vi "cRIO_onboard_laser_log.vi"() -> ()   [LabVIEW 2020]
uses:
  <vilib>/Platform/TimedLoop/XDataNode/timing_clust.ctl
  <vilib>/Platform/TimedLoop/XDataNode/nitl_modes.ctl
  <vilib>/Platform/TimedLoop/XDataNode/wakeup.ctl
  <vilib>/Utility/file.llb/Write Delimited Spreadsheet (DBL).vi
  <vilib>/Platform/TimedLoop/XDataNode/loadnilvce.vi
  <vilib>/platform/TimedLoop/XDataNode/XDataNode.xnode
  <vilib>/Platform/TimedLoop/XDataNode/XDNodeRunTimeDep.lvlib
panel:
  out "Laser Displacement - cRIO (onboard execution)":dbl[][](graph)
  out "Readout (V)":dbl[][](array[numeric])
  in  "Log Data":bool
  out "Laser Displacement - cRIO (logged data)":dbl[][](graph)
  in  "stop":bool
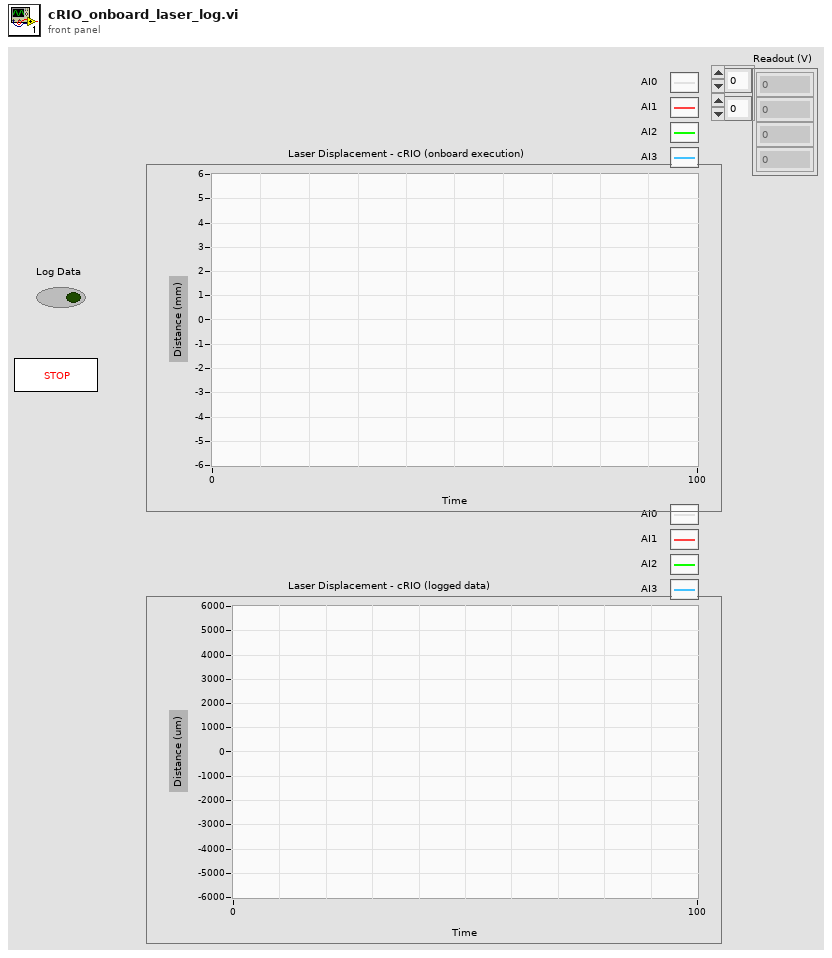
[diagram p1: front panel]
types:
  T1 = typedef "XDNodeRunTimeDep.lvlib/timing_clust.ctl" = cluster{"Expected End [f-1]":u64, "Actual End [f-1]":u64, "Finished Late? [f-1]":bool, "Expected End [i-1]":u64, "Actual End [i-1]":u64, "Finished Late? [i-1]":bool, "Expected Start [i]":u64, "Actual Start [i]":u64, "Expected Start [f]":u64, "Actual Start [f]":u64, "Source Name":string, "Structure Name":string, "Period":i64, "Deadline":i64, "Offset":i64, "Start":i64, "Priority":i32, "Timeout":i32, "Mode":T2, "Wakeup Reason":T3, "Error":errorcluster, "Source Type":string, "Secondary Source Type":string, "Global End Time":u64, "Global Start Time":u64, "Frame Duration":u64, "Iteration Duration":u64, "Assigned CPU":i32, "I/O Scan Engine Mode":u32}
  T2 = typedef "XDNodeRunTimeDep.lvlib/nitl_modes.ctl" = enum32{"No Change", "Process missed periods, maintain original phase", "Discard missed periods, maintain original phase", "Process missed periods, ignore original phase", "Discard missed periods, ignore original phase"}
  T3 = typedef "XDNodeRunTimeDep.lvlib/wakeup.ctl" = enum32{"Normal", "Aborted", "Asynchronous wakeup", "Timing source error", "Timed loop error", "Timeout"}
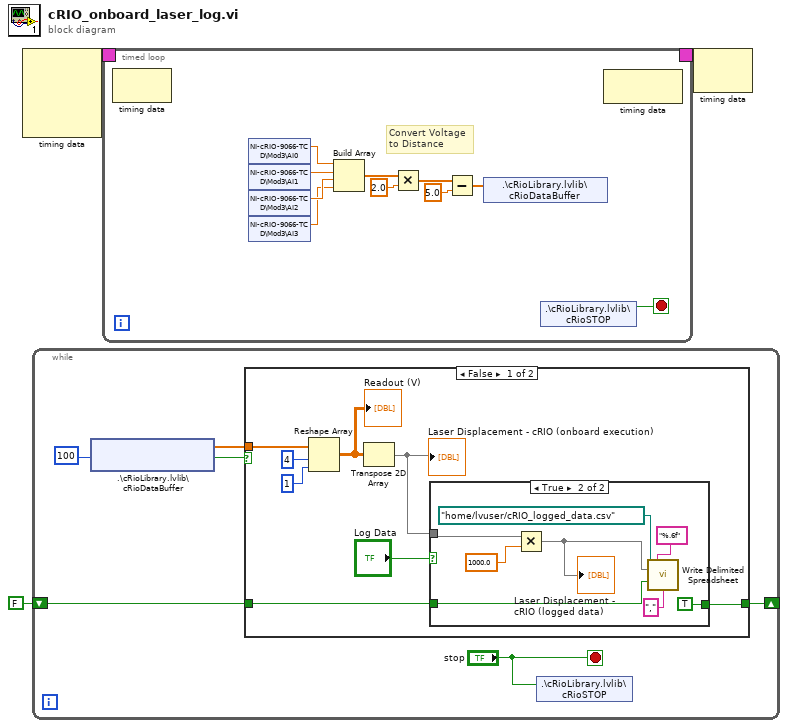
[diagram p0: block diagram]
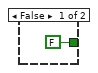
[diagram p2: hidden frame]
diagram:
  n1 = node-c288() -> (w3:T1)  [unwired: 4 in]
  n2 = while {
    shift-right: [w9] -> _
    shift-left: FALSE -> [w8]
    stop <- "stop" stop-if-true
    n3 = shared-variable ".\\cRioLibrary.lvlib\\cRioDataBuffer"(100) -> (w6:dbl[], w5:bool)  [unwired: 1 in, 1 out]
    n4 = case shown="False" w5 {
      tunnel: w6 -> [w11 _]
      tunnel: [w12 w27] -> w9
      tunnel: w8 -> [w17 w27]
      frame False {
        n5 = Reshape Array(w11, 4 ("dimension size"), 1 ("dimension size")) -> (w14:dbl[][])
        "Readout (V)" <- w14
        n6 = Transpose 2D Array(2D array=w14) -> (transposed array=w10:dbl[][])
        "Laser Displacement - cRIO (onboard execution)" <- w10
        n7 = case shown="True" "Log Data" {
          tunnel: w17 -> [_ w21]
          tunnel: w10 -> [_ w25]
          tunnel: [FALSE TRUE] -> w12
          frame False {
          }
          frame True {
            n8 = Multiply(x=w25, y=1000.0) -> (x*y=w19:dbl[][])
            "Laser Displacement - cRIO (logged data)" <- w19
            n9 = call-poly <vilib>:"Write Delimited Spreadsheet.vi"("file path (dialog if empty)"=path "/home/lvuser/cRIO_logged_data.csv", "format (%.3f)"="%.6f", "2D data"=w19, "append to file? (new file:F)"=w21, "delimiter (\\t)"="," ("delimiter (\\t)")) -> ()  [unwired: 9 in, 2 out]
          }
        }
      }
      frame True {
      }
    }
    n10 = shared-variable ".\\cRioLibrary.lvlib\\cRioSTOP"("stop") -> ()  [unwired: 1 in, 1 out]
  }
  n11 = timed-loop {
    timing: w3 -> [_]
    timing-out: [_] -> w2
    stop <- w37 stop-if-true
    # "Convert Voltage to Distance"
    n12 = node-c288() -> ()  [unwired: 1 in, 1 out]
    n13 = shared-variable "NI-cRIO-9066-TCD\\Mod3\\AI0"() -> (w33:dbl)  [unwired: 1 in, 1 out]
    n14 = shared-variable "NI-cRIO-9066-TCD\\Mod3\\AI1"() -> (w30:dbl)  [unwired: 1 in, 1 out]
    n15 = shared-variable "NI-cRIO-9066-TCD\\Mod3\\AI2"() -> (w32:dbl)  [unwired: 1 in, 1 out]
    n16 = shared-variable "NI-cRIO-9066-TCD\\Mod3\\AI3"() -> (w31:dbl)  [unwired: 1 in, 1 out]
    n17 = Build Array(w33, w30, w32, w31) -> (w28:dbl[])
    n18 = Multiply(x=w28, y=2.0) -> (x*y=w35:dbl[])
    n19 = Subtract(x=w35, y=5.0) -> (x-y=w29:dbl[])
    n20 = shared-variable ".\\cRioLibrary.lvlib\\cRioDataBuffer"(w29) -> ()  [unwired: 1 in, 1 out]
    n21 = shared-variable ".\\cRioLibrary.lvlib\\cRioSTOP"() -> (w37:bool)  [unwired: 1 in, 1 out]
    n22 = node-c288() -> ()  [unwired: 1 in, 1 out]
  }
  n23 = node-c288(w2) -> ()  [unwired: 1 out]
